vi "counter read.vi"(0 "connection reference":T2, 4 "DB write":T1, 5 "error in (no error)":errorcluster, 7 "Enter Part Unique id":string="A1234567B567", 8 "search dataString":string, 11 "Enum":enum16{"Write", "Read"}(ring)=enum."Read") -> (14 "connection reference out":T2, 15 "last id":variant[][](array[variant]), 16 "Search result":string[][](table), 17 "DMC TESTED:T":bool, 19 "error out":errorcluster)   [LabVIEW 2015]
uses:
  <vilib>/addons/database/NI_Database_API.lvlib
  <vilib>/addons/database/_DB Variant To Data/Database Variant To Data.xnode
  <vilib>/addons/database/Connection.llb/Conn ObjectReference.ctl
panel:
  out "columns":string[](array[string])
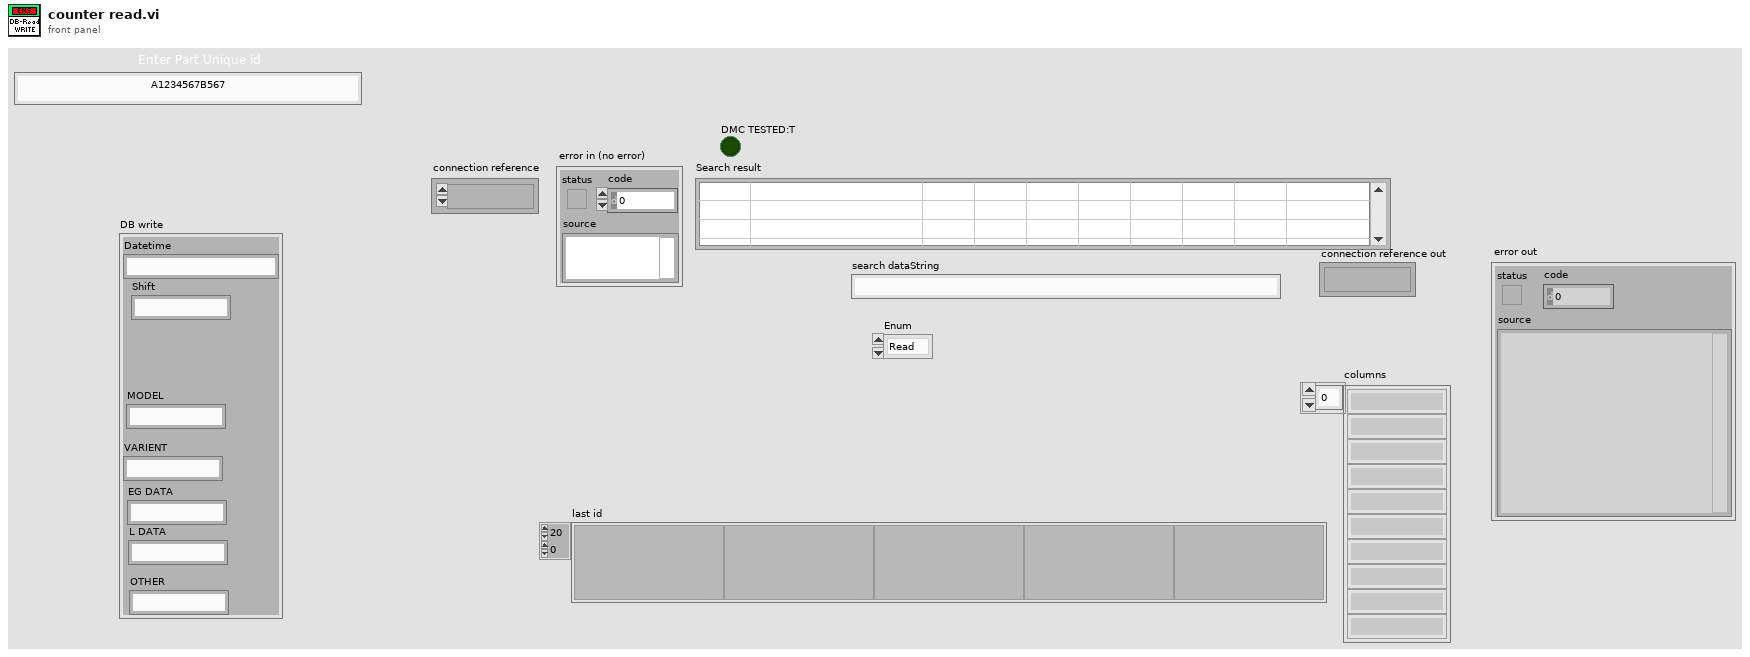
[diagram p1: front panel]
types:
  T1 = cluster{"Datetime":string, "Shift":string, "MODEL":string, "VARIENT":string, "EG DATA":string, "L DATA":string, "OTHER":string}
  T2 = typedef "NI_Database_API.lvlib/Conn ObjectReference.ctl" = refnum<k1>
  T3 = cluster{"DATETIME":string, "MODELNAME":string, "BARCODE":string, "MARK":string, "OTHER":string}
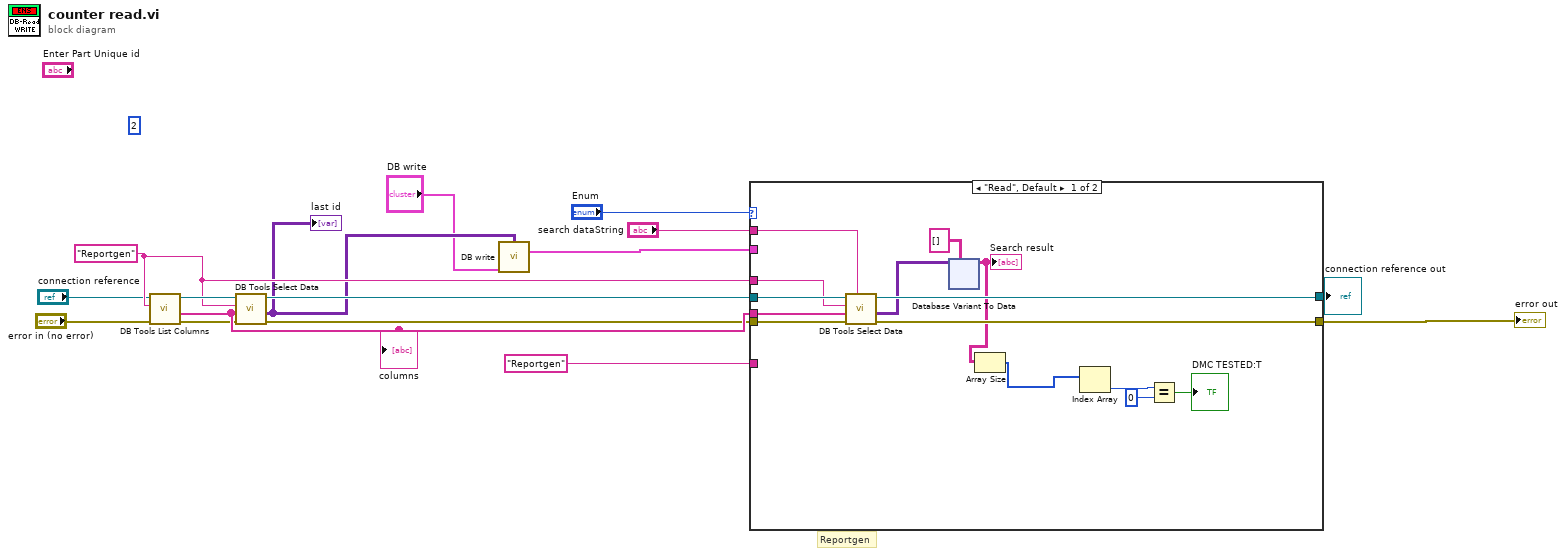
[diagram p0: block diagram]
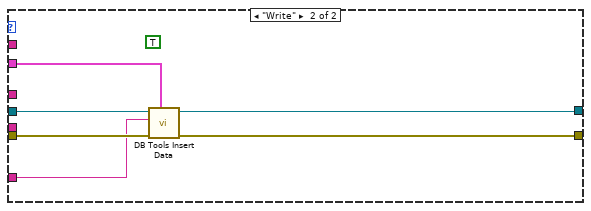
[diagram p2: hidden frame]
diagram:
  (unwired) i16 2 ("precision (6)")
  w9 = "Reportgen" ("table")
  # "Reportgen"
  n1 = call <vilib>:"DB Tools List Columns.vi"("error in (no error)"="error in (no error)", "table"=w9, "connection reference"="connection reference") -> ("error out"=w14:errorcluster, "columns"=w16:string[], "connection reference out"=w15:T2)  [unwired: 1 in, 1 out]
  "columns" <- w16
  n2 = call <vilib>:"DB Tools Select Data.vi"("error in (no error)"=w14, "columns"=w16, "table"=w9, "connection reference"=w15) -> ("error out"=w13:errorcluster, "data"=w3:variant[][], "connection reference out"=w12:T2)  [unwired: 2 in]
  "last id" <- w3
  n3 = call "DB write.vi"("DB data"=w3, "DB write"="DB write") -> ("DB write"=w2:T3)  [unwired: 13 in]
  n4 = case shown="\"Read\", Default" "Enum" {
    tunnel: [w26 w80] -> w4
    tunnel: [w25 w79] -> w5
    tunnel: w16 -> [w27 _]
    tunnel: w13 -> [w29 w78]
    tunnel: w12 -> [w30 w77]
    tunnel: "Reportgen" ("table") -> [_ w76]
    tunnel: w9 -> [w28 _]
    tunnel: w2 -> [_ w75]
    tunnel: "search dataString" -> [w24 _]
    frame "Read", Default {
      n5 = call <vilib>:"DB Tools Select Data.vi"("condition"=w24, "error in (no error)"=w29, "columns"=w27, "table"=w28, "connection reference"=w30) -> ("error out"=w25:errorcluster, "data"=w22:variant[][], "connection reference out"=w26:T2)  [unwired: 1 in]
      n6 = xnode "Database Variant To Data"("database variant"=w22, "type"=string[][] [] ("Array")) -> ("data"=w21:string[][])  [unwired: 1 in, 1 out]
      "Search result" <- w21
      n7 = Array Size(array=w21) -> (size(s)=w20:i32[])
      n8 = Index Array(array=w20) -> (element=w19:i32)  [unwired: 1 in]
      n9 = Equal?(x=w19, y=0) -> (x = y?=→"DMC TESTED:T":bool)
    }
    frame "Write" {
      (unwired) TRUE ("create table? (F)")
      n10 = call <vilib>:"DB Tools Insert Data.vi"("data"=w75, "error in (no error)"=w78, "table"=w76, "connection reference"=w77) -> ("error out"=w79:errorcluster, "connection reference out"=w80:T2)  [unwired: 6 in]
    }
  }
  "error out" <- w5
  "connection reference out" <- w4
